vi "SAOMM-Graph-Hexapode.vi"(0 "Hexapod cluster":T1 {"Hexapode_ServoY" format="%.6f"; "Hexapod_Console" format="%.6f"; "Hexapod_Position" format="%.6f"}, 1 "LoggingTimeStamp":dbl, 2 "DataLenght (seconds)":dbl, 7 "X IN":cluster{dbl[], dbl[]}[](array[cluster]) {"?" format="%.3f"}, 9 "Y IN":cluster{dbl[], dbl[]}[](array[cluster]) {"?" format="%.3f"}, 11 "Cumul IN":cluster{dbl[], dbl[]}[](array[cluster]) {"?" format="%.3f"}) -> (8 "X OUT":cluster{dbl[], dbl[]}[](array[cluster]) {"?" format="%.3f"}, 10 "Y OUT":cluster{dbl[], dbl[]}[](array[cluster]) {"?" format="%.3f"}, 15 "Cumul OUT":cluster{dbl[], dbl[]}[](array[cluster]) {"?" format="%.3f"})   [LabVIEW 2011]
panel:
  out "Activité":bool
  out "CumY":dbl format="%.6f"
  out "CumX":dbl format="%.6f"
  out "ErrY":dbl format="%.6f"
  out "ErrX":dbl format="%.6f"
  out "Index of Treshold":dbl
  out "CurrentTimeStamp":dbl format="%.3f"
  out "CmdY":dbl format="%.6f"
  out "CmdX":dbl format="%.6f"
  out "HexY":dbl format="%.6f"
  out "HexX":dbl format="%.6f"
  out "TimeStampTreshold":dbl format="%.3f"
  # "Variables intermédiaire"
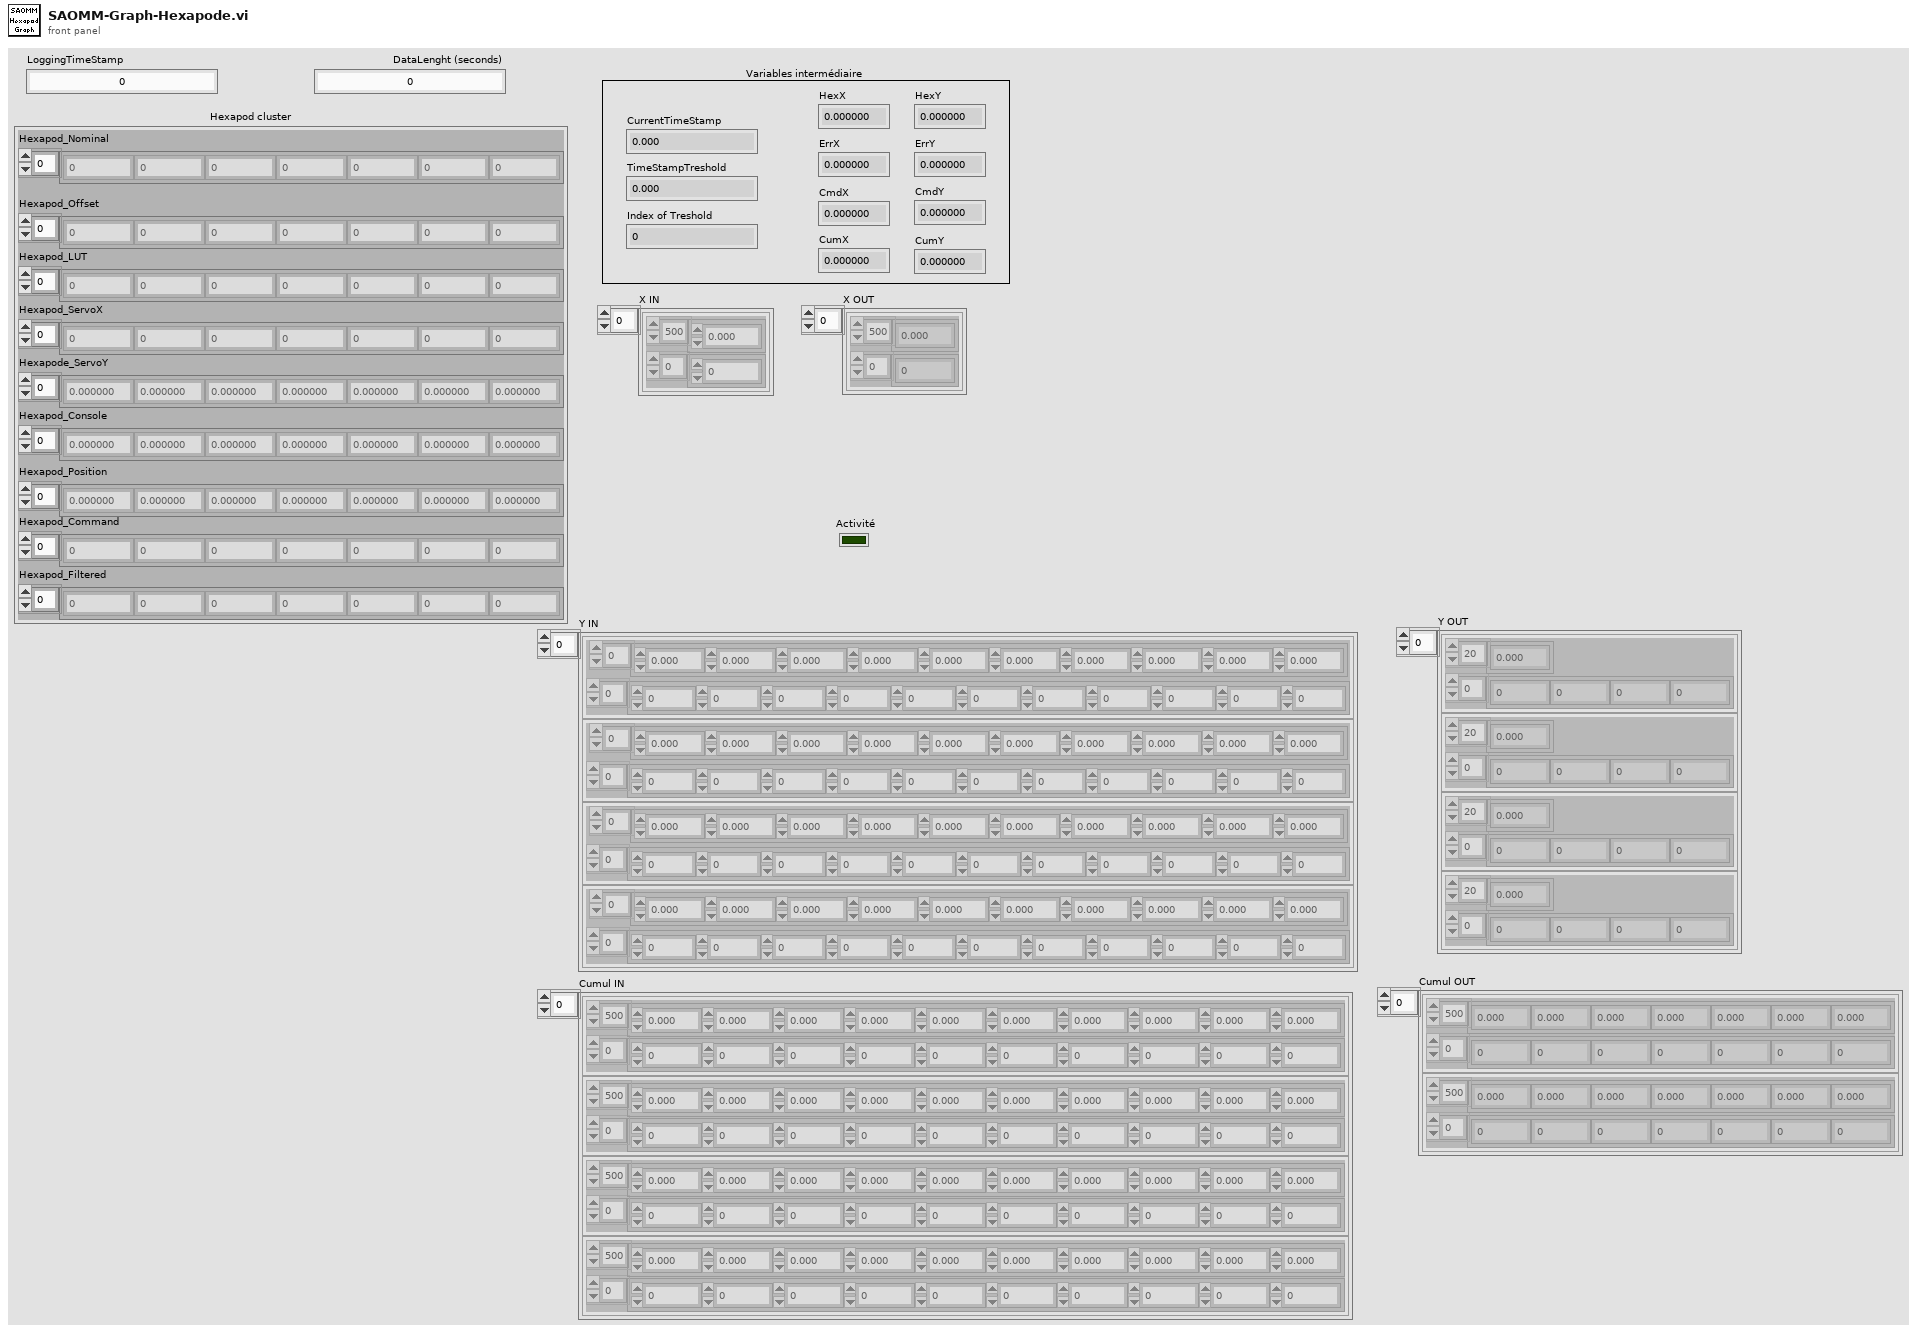
[diagram p1: front panel]
types:
  T1 = cluster{"Hexapod_Nominal":dbl[], "Hexapod_Offset":dbl[], "Hexapod_LUT":dbl[], "Hexapod_ServoX":dbl[], "Hexapode_ServoY":dbl[], "Hexapod_Console":dbl[], "Hexapod_Position":dbl[], "Hexapod_Command":dbl[], "Hexapod_Filtered":dbl[]}
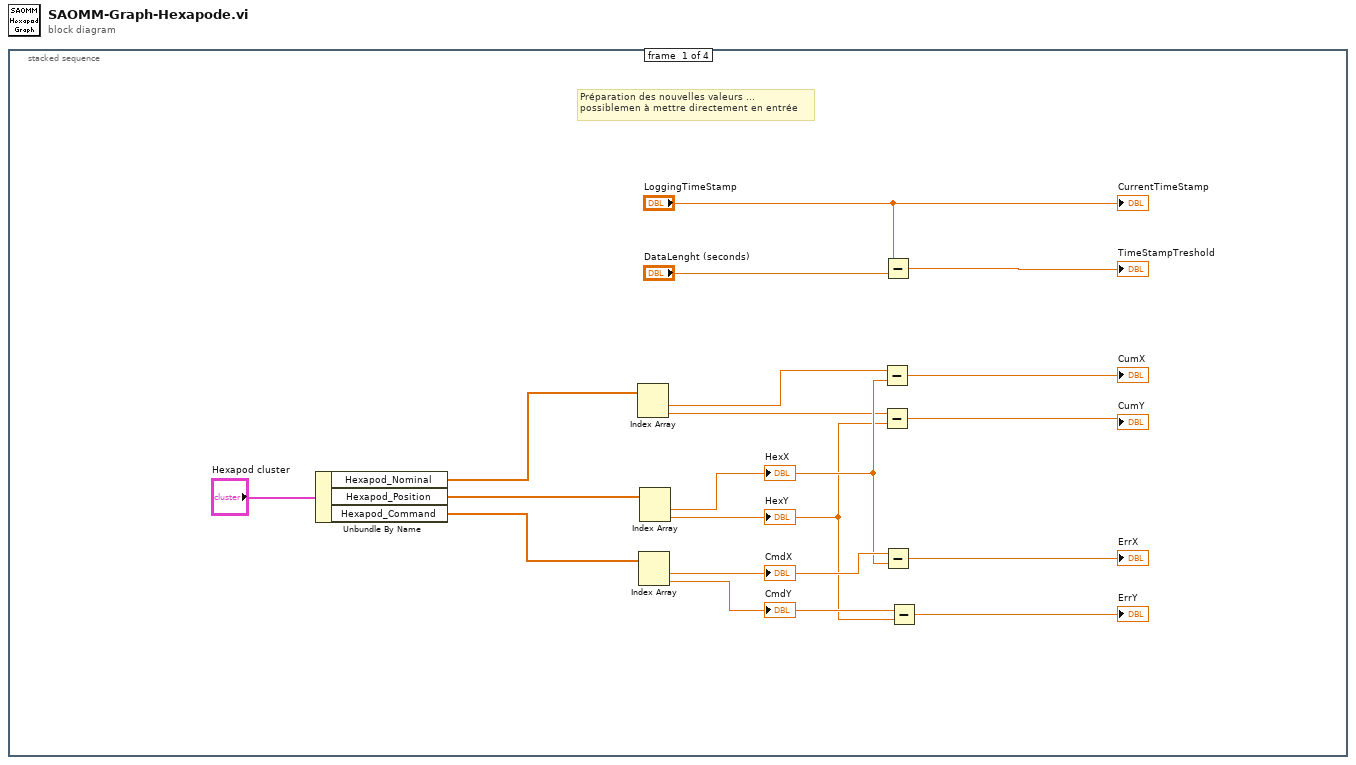
[diagram p0: block diagram]
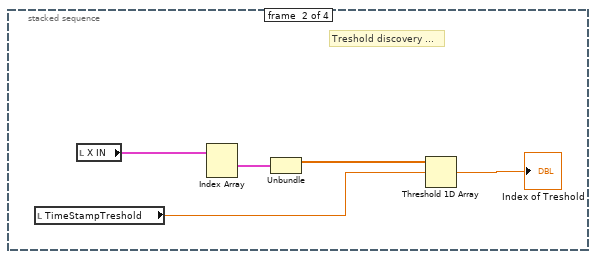
[diagram p2: hidden frame]
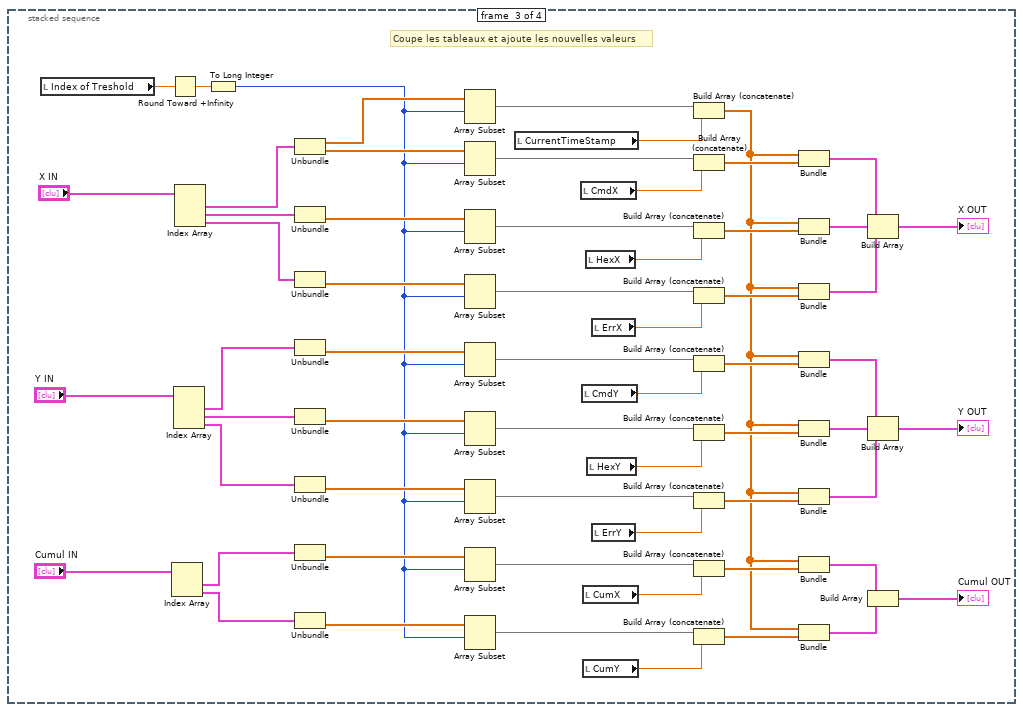
[diagram p3: hidden frame]
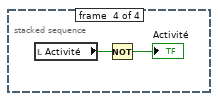
[diagram p4: hidden frame]
diagram:
  n1 = stacked-sequence {
    frame #0 {
      # "Préparation des nouvelles valeurs ...\npossiblemen à mettre directement en entrée"
      n2 = Unbundle By Name("Hexapod cluster") -> ("Hexapod_Nominal"=w8:dbl[], "Hexapod_Position"=w13:dbl[], "Hexapod_Command"=w14:dbl[])
      n3 = Index Array(array=w8) -> (element #1=w3:dbl, element #2=w2:dbl)  [unwired: 2 in]
      n4 = Index Array(array=w14) -> (element #1=w12:dbl, element #2=w11:dbl)  [unwired: 2 in]
      "CmdX" <- w12
      "CmdY" <- w11
      n5 = Index Array(array=w13) -> (element #1=w5:dbl, element #2=w4:dbl)  [unwired: 2 in]
      "HexY" <- w4
      "HexX" <- w5
      n6 = Subtract(x=w3, y=w5) -> (x-y=→"CumX":dbl)
      n7 = Subtract(x=w2, y=w4) -> (x-y=→"CumY":dbl)
      n8 = Subtract(x="LoggingTimeStamp", y="DataLenght (seconds)") -> (x-y=→"TimeStampTreshold":dbl)
      n9 = Subtract(x=w12, y=w5) -> (x-y=→"ErrX":dbl)
      n10 = Subtract(x=w11, y=w4) -> (x-y=→"ErrY":dbl)
      "CurrentTimeStamp" <- "LoggingTimeStamp"
    }
    frame #1 {
      # "Treshold discovery ..."
      n11 = local read "TimeStampTreshold"() -> (w20:dbl)
      n12 = local read "X IN"() -> (w21:cluster{dbl[], dbl[]}[])
      n13 = Index Array(array=w21) -> (element #1=w22:cluster{dbl[], dbl[]})  [unwired: 2 in, 1 out]
      n14 = Unbundle(w22) -> (w19:dbl[])  [unwired: 1 out]
      n15 = Threshold 1D Array(2:w20, 3:w19) -> (0:→"Index of Treshold":dbl)  [unwired: 1 in]
    }
    frame #2 {
      # "Coupe les tableaux et ajoute les nouvelles valeurs"
      n16 = local read "Index of Treshold"() -> (w64:dbl)
      n17 = Round Toward +Infinity(x=w64) -> (ceil(x): smallest int >= x=w63:dbl)
      n18 = Index Array(array="Cumul IN") -> (element #1=w78:cluster{dbl[], dbl[]}, element #2=w77:cluster{dbl[], dbl[]})  [unwired: 2 in]
      n19 = Index Array(array="Y IN") -> (element #1=w42:cluster{dbl[], dbl[]}, element #2=w79:cluster{dbl[], dbl[]}, element #3=w80:cluster{dbl[], dbl[]})  [unwired: 3 in]
      n20 = Index Array(array="X IN") -> (element #1=w82:cluster{dbl[], dbl[]}, element #2=w81:cluster{dbl[], dbl[]}, element #3=w44:cluster{dbl[], dbl[]})  [unwired: 3 in]
      n21 = To Long Integer(number=w63) -> (32bit integer=w31:i32)
      n22 = Unbundle(w82) -> (w62:dbl[], w61:dbl[])
      n23 = Unbundle(w81) -> (w60:dbl[])  [unwired: 1 out]
      n24 = Unbundle(w44) -> (w46:dbl[])  [unwired: 1 out]
      n25 = Unbundle(w42) -> (w45:dbl[])  [unwired: 1 out]
      n26 = Unbundle(w79) -> (w59:dbl[])  [unwired: 1 out]
      n27 = Unbundle(w80) -> (w58:dbl[])  [unwired: 1 out]
      n28 = Unbundle(w78) -> (w57:dbl[])  [unwired: 1 out]
      n29 = Unbundle(w77) -> (w34:dbl[])  [unwired: 1 out]
      n30 = Array Subset(array=w62, index=w31) -> (w51:dbl[])  [unwired: 1 in]
      n31 = Array Subset(array=w61, index=w31) -> (w56:dbl[])  [unwired: 1 in]
      n32 = Array Subset(array=w60, index=w31) -> (w55:dbl[])  [unwired: 1 in]
      n33 = Array Subset(array=w46, index=w31) -> (w48:dbl[])  [unwired: 1 in]
      n34 = Array Subset(array=w45, index=w31) -> (w47:dbl[])  [unwired: 1 in]
      n35 = Array Subset(array=w59, index=w31) -> (w54:dbl[])  [unwired: 1 in]
      n36 = Array Subset(array=w58, index=w31) -> (w53:dbl[])  [unwired: 1 in]
      n37 = Array Subset(array=w57, index=w31) -> (w52:dbl[])  [unwired: 1 in]
      n38 = Array Subset(array=w34, index=w31) -> (w35:dbl[])  [unwired: 1 in]
      n39 = local read "CurrentTimeStamp"() -> (w65:dbl)
      n40 = local read "CmdX"() -> (w66:dbl)
      n41 = local read "CmdY"() -> (w40:dbl)
      n42 = local read "CumX"() -> (w68:dbl)
      n43 = local read "CumY"() -> (w67:dbl)
      n44 = local read "HexX"() -> (w36:dbl)
      n45 = local read "HexY"() -> (w37:dbl)
      n46 = local read "ErrX"() -> (w41:dbl)
      n47 = local read "ErrY"() -> (w39:dbl)
      n48 = Build Array (concatenate)(w51, w65) -> (w23:dbl[])
      n49 = Build Array (concatenate)(w56, w66) -> (w26:dbl[])
      n50 = Build Array (concatenate)(w55, w36) -> (w25:dbl[])
      n51 = Build Array (concatenate)(w48, w41) -> (w49:dbl[])
      n52 = Build Array (concatenate)(w47, w40) -> (w50:dbl[])
      n53 = Build Array (concatenate)(w54, w37) -> (w24:dbl[])
      n54 = Build Array (concatenate)(w53, w39) -> (w70:dbl[])
      n55 = Build Array (concatenate)(w52, w68) -> (w69:dbl[])
      n56 = Build Array (concatenate)(w35, w67) -> (w33:dbl[])
      n57 = Bundle(w23, w26) -> (w76:cluster{dbl[], dbl[]})  [unwired: 1 in]
      n58 = Bundle(w23, w25) -> (w75:cluster{dbl[], dbl[]})  [unwired: 1 in]
      n59 = Bundle(w23, w49) -> (w43:cluster{dbl[], dbl[]})  [unwired: 1 in]
      n60 = Bundle(w23, w50) -> (w38:cluster{dbl[], dbl[]})  [unwired: 1 in]
      n61 = Bundle(w23, w24) -> (w74:cluster{dbl[], dbl[]})  [unwired: 1 in]
      n62 = Bundle(w23, w70) -> (w73:cluster{dbl[], dbl[]})  [unwired: 1 in]
      n63 = Bundle(w23, w69) -> (w72:cluster{dbl[], dbl[]})  [unwired: 1 in]
      n64 = Bundle(w23, w33) -> (w71:cluster{dbl[], dbl[]})  [unwired: 1 in]
      n65 = Build Array(w76, w75, w43) -> (→"X OUT":cluster{dbl[], dbl[]}[])
      n66 = Build Array(w38, w74, w73) -> (→"Y OUT":cluster{dbl[], dbl[]}[])
      n67 = Build Array(w72, w71) -> (→"Cumul OUT":cluster{dbl[], dbl[]}[])
    }
    frame #3 {
      n68 = local read "Activité"() -> (w85:bool)
      n69 = Not(x=w85) -> (.not. x?=→"Activité":bool)
    }
  }
